vi "Calculatrice.vi"() -> ()   [LabVIEW 2020]
panel:
  in  "Btn_Error":bool caption="Error"
  out "sortie d'erreur":errorcluster
  in  "Btn_Stop":bool
  out "Display":cluster{"Num":dbl, "Char":string}
  in  "Pad":T1
  # "Calculatrice"
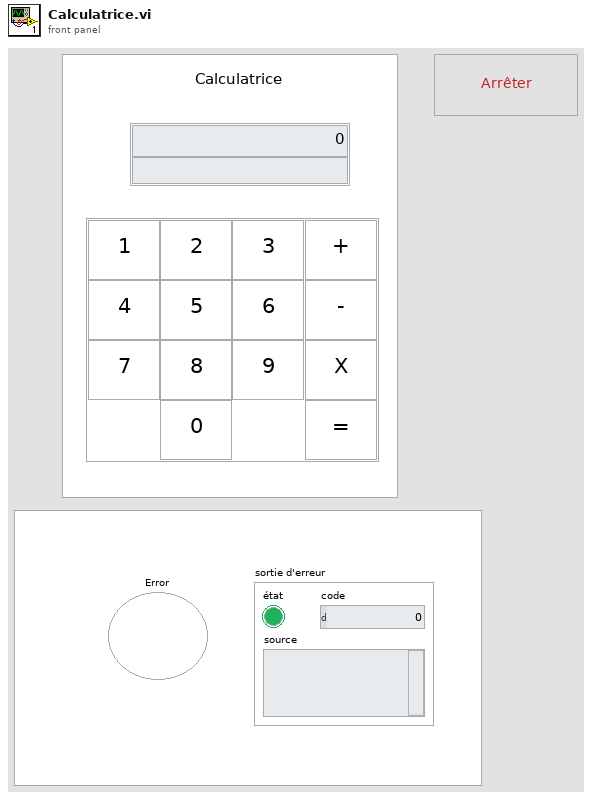
[diagram p1: front panel]
types:
  T1 = cluster{"Btn_1":bool, "Btn_2":bool, "Btn_3":bool, "Btn_4":bool, "Btn_5":bool, "Btn_6":bool, "Btn_7":bool, "Btn_8":bool, "Btn_9":bool, "Btn_0":bool, "Btn_+":bool, "Btn_-":bool, "Btn_X":bool, "Btn_=":bool}
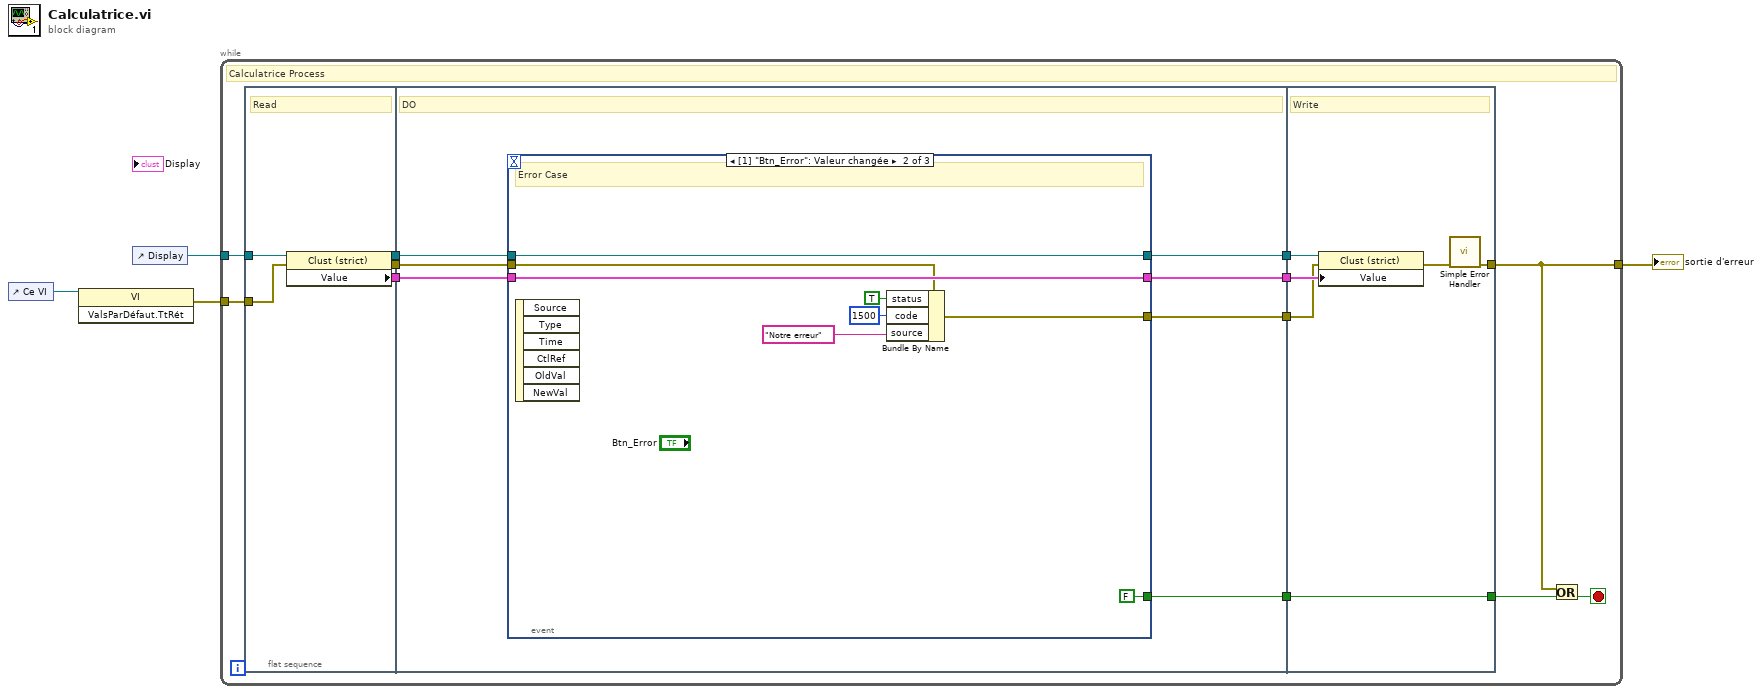
[diagram p0: block diagram]
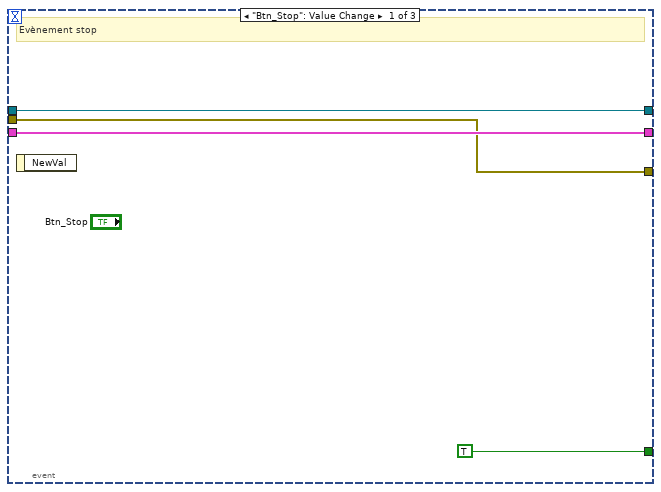
[diagram p2: hidden frame]
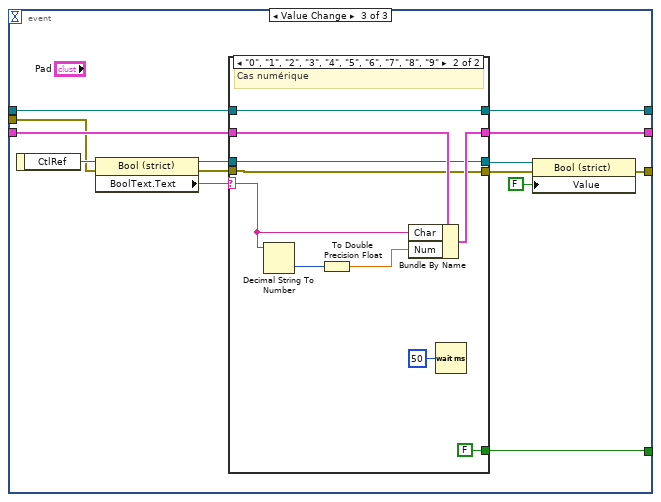
[diagram p3: hidden frame]
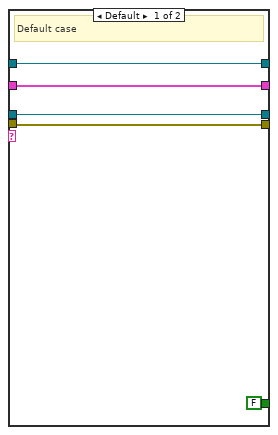
[diagram p4: hidden frame]
diagram:
  n1 = control-ref of="Ce VI"() -> (w3:refnum<vi>)
  n2 = invoke class="VI" method="ValsParDéfaut.TtRét"(reference=w3) -> (error out=w2:errorcluster)  [unwired: 2 in, 2 out]
  n3 = control-ref of="Display"() -> (w4:refnum<vi>)
  n4 = while {
    tunnel: w4 -> [w14]
    tunnel: w2 -> [w9]
    tunnel: [w5] -> w1
    stop <- w6 stop-if-true
    # "Calculatrice Process"
    n5 = flat-sequence {
      tunnel: w14 -> [w21]
      tunnel: [w20] -> w13
      tunnel: [w19] -> w12
      tunnel: w9 -> [w17]
      tunnel: [w18] -> w8
      tunnel: [w28] -> w15
      tunnel: w13 -> [w27]
      tunnel: w12 -> [w26]
      tunnel: [w25] -> w11
      tunnel: [w24] -> w10
      tunnel: w8 -> [w23]
      tunnel: [w22] -> w7
      tunnel: [w75] -> w16
      tunnel: w15 -> [w75]
      tunnel: w11 -> [w74]
      tunnel: w10 -> [w73]
      tunnel: w7 -> [w72]
      tunnel: [w70] -> w5
      frame #0 {
        # "Read"
        n6 = property class="Clust (strict)"(reference=w21, error in=w17) -> (reference out=w19:refnum<vi>, error out=w18:errorcluster, "Value"=w20:cluster{"Num":dbl, "Char":string})
      }
      frame #1 {
        # "DO"
        n7 = event shown="[1] \"Btn_Error\": Valeur changée" {
          selector: _ -> [_ _ _]
          dyn-events: _ -> [_ _ _]
          timeout: _ -> [_ _ _]
          tunnel: [TRUE FALSE w52] -> w28
          tunnel: w27 -> [w30 w38 w51]
          tunnel: w26 -> [w31 w39 w50]
          tunnel: [w31 w39 w49] -> w25
          tunnel: [w30 w38 w48] -> w24
          tunnel: w23 -> [w29 w37 w44]
          tunnel: [w29 w36 w41] -> w22
          event "Btn_Stop": Value Change {
            # "Evènement stop"
            n8 = event-data() -> ()  [unwired: 1 in, 1 out]
          }
          event "Btn_Error": Value Change {
            # "Error Case"
            n9 = event-data() -> ()  [unwired: 1 in, 6 out]
            n10 = Bundle By Name(cluster=w37, "status"=TRUE, "code"=1500, "source"="Notre erreur") -> (w36:errorcluster)
          }
          event "Pad.Btn_1", "Pad.Btn_2", "Pad.Btn_3", "Pad.Btn_4", "Pad.Btn_5", "Pad.Btn_6", "Pad.Btn_7", "Pad.Btn_8", "Pad.Btn_9", "Pad.Btn_0": Value Change {
            n11 = event-data() -> ("CtlRef"=w54:refnum<vi>)  [unwired: 1 in]
            n12 = property class="Bool (strict)"(reference=w54, error in=w44) -> (reference out=w47:refnum<vi>, error out=w43:errorcluster, "BoolText.Text"=w53:string)
            n13 = case shown="\"0\", \"1\", \"2\", \"3\", \"4\", \"5\", \"6\", \"7\", \"8\", \"9\"" w53 {
              selector: w53 -> [_ w63]
              tunnel: [FALSE FALSE] -> w52
              tunnel: w51 -> [w57 w67]
              tunnel: w50 -> [w58 w68]
              tunnel: [w58 w68] -> w49
              tunnel: [w57 w66] -> w48
              tunnel: w47 -> [w56 w65]
              tunnel: [w56 w65] -> w46
              tunnel: w43 -> [w55 w60]
              tunnel: [w55 w60] -> w42
              frame Default {
                # "Default case"
              }
              frame "0", "1", "2", "3", "4", "5", "6", "7", "8", "9" {
                # "Cas numérique"
                n14 = Decimal String To Number(string=w63) -> (number=w62:i32)  [unwired: 2 in, 1 out]
                n15 = To Double Precision Float(number=w62) -> (double precision float=w61:dbl)
                n16 = Bundle By Name(cluster=w67, "Char"=w63, "Num"=w61) -> (w66:cluster{"Num":dbl, "Char":string})
                n17 = Wait (ms)(milliseconds to wait=u32 50 ("attente (ms)")) -> ()  [unwired: 1 out]
              }
            }
            n18 = property class="Bool (strict)"(reference=w46, error in=w42, "Value"=FALSE ("Valeur")) -> (error out=w41:errorcluster)  [unwired: 1 out]
          }
        }
      }
      frame #2 {
        # "Write"
        n19 = property class="Clust (strict)"(reference=w74, error in=w72, "Value"=w73) -> (error out=w71:errorcluster)  [unwired: 1 out]
        n20 = call <vilib>:"Simple Error Handler.vi"("error in (no error)"=w71) -> ("error out"=w70:errorcluster)  [unwired: 4 in, 4 out]
      }
    }
    n21 = Or(x=w5, y=w16) -> (x .or. y?=w6:bool)
  }
  "sortie d'erreur" <- w1
